vi "IR_analog_to_digital.vi"(9 "logic_num":dbl, 10 "IR_IN":dbl) -> (2 "IR_OUT":bool)   [LabVIEW 2017]
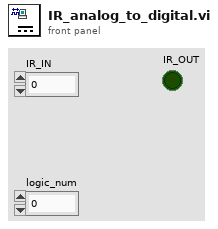
[diagram p1: front panel]
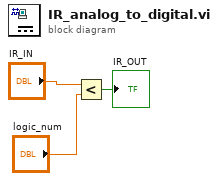
[diagram p0: block diagram]
diagram:
  n1 = Less?(x="IR_IN", y="logic_num") -> (x < y?=→"IR_OUT":bool)
